vi "Configure.vi"(8 "error in":errorcluster, 10 "name":string="nCRDS", 11 "nCRD in":refnum<class "nCRD.lvclass">) -> (0 "error out":errorcluster, 3 "nCRD out":refnum<class "nCRD.lvclass">)   [LabVIEW 2015, in "nCRD.lvclass"]
doc: "Configures the CRDS for operation and starts all DAQmx tasks associated with the instrument. This VI overrides the parent VI in the Instrument class."
uses:
  nCRD.lvclass
  Reusable/Instrument/state.ctl
  Session/Raw FPGA/FPGA Session.lvclass
  nCRD.lvclass/nCRD.ctl
  Session/Raw FPGA/FPGA Session.lvclass/FPGA Session.ctl
  Reusable/Instrument/Instrument.lvclass/Instrument.ctl
  Session/Raw FPGA/Read FPGA Ref.vi
  Accessors/Write RepRate.vi
  Accessors/Write SamplesPerCycle.vi
  Reusable/Instrument/Read Log Session.vi
  <vilib>/Utility/error.llb/Error Cluster From Error Code.vi
  <vilib>/rvi/errors/niLvFpgaAdjustHostInterfaceError.vi
  Reusable/CRDS/Main/Read Cells.vi
  Reusable/CRDS/Cell/Write dt.vi
  Reusable/CRDS/Main/Write Cells.vi
  <vilib>/rvi/interface/common/niFpgaWaitOnOcc.vi
  FPGA Ref.ctl
  <vilib>/rvi/interface/nirviReadWriteControl/nirviReadWriteControl.xnode
  FPGA Bitfiles/NickIO.lvbitx
  Reusable/CRDS/Cell/CRDS Cell.lvclass
  <userlib>/_Session Fwk/Session - Root.lvclass
  <vilib>/rvi/interface/nirviMethod/nirviMethod.xnode
  Reusable/CRDS/Main/CRDS.lvclass
  <vilib>/rvi/errors/niLvFpgaMergeErrorWithErrorCode.vi
  Reusable/Instrument/Instrument.lvclass
  Reusable/Session Log/System Log.lvclass
  NiFpgaLv.dll
  <vilib>/FPGAPlugInAG/cRIO-9081/niLvFpga_ConfigureFifo_cRIO-9081.vi
  <vilib>/FPGAPlugInAG/cRIO-9081/niLvFpga_StartFifo_cRIO-9081.vi
panel:
  out "Actual Depth":u32
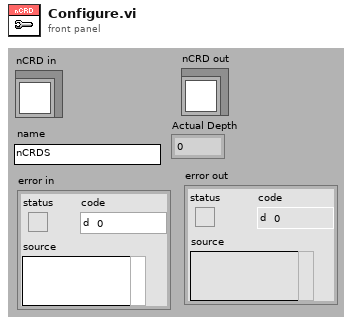
[diagram p1: front panel]
types:
  T1 = typedef "Instrument.lvclass/state.ctl" = enum8{"Configure", "Acquire", "Wait", "Quit", "Handle Error", "NOOP"}
  T2 = typedef "Session - Root.lvclass/Session Handle.ctl" = refnum<data-value>
  T3 = typedef "FPGA Ref.ctl" = refnum<k20>
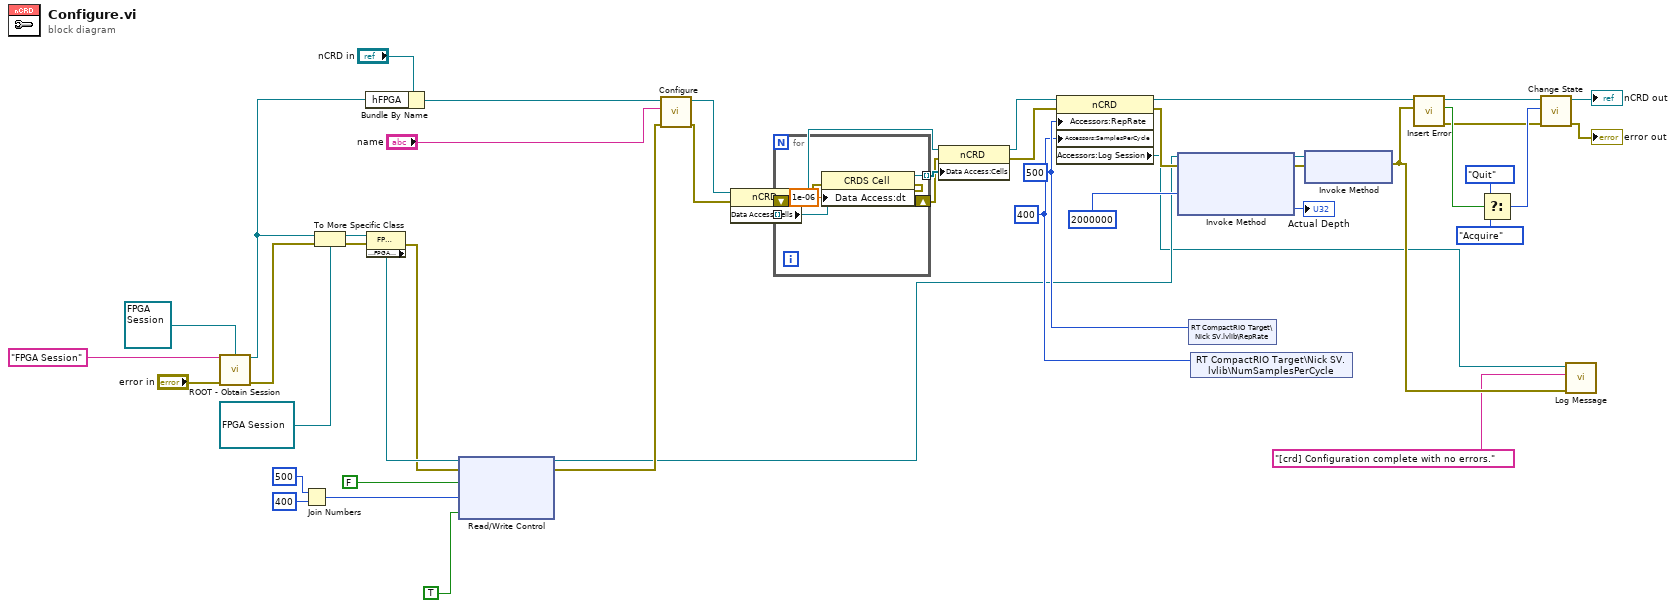
[diagram p0: block diagram]
diagram:
  w43 = u16 400 ("SamplesPerCycle")
  w44 = u16 500 ("RepRate")
  n1 = call <userlib>:"ROOT - Obtain Session.vi"("Session Name ()"="FPGA Session", "OBJ - Session"=refnum<class "FPGA Session.lvclass"> refnum ("FPGA Session.lvclass"), "error in (no error)"="error in") -> ("Session Handle"=w21:T2, "error out"=w20:errorcluster)  [unwired: 10 in, 1 out]
  n2 = Join Numbers(hi=u16 500 ("NumSamples"), lo=u16 400 ("DutyCycle")) -> ((hi.lo)=w1:u32)
  n3 = To More Specific Class(target class=refnum<data-value> refnum ("hFPGA"), reference=w21, error in=w20) -> (specific class reference=w28:refnum<data-value>, error out=w19:errorcluster)
  n4 = Bundle By Name(cluster="nCRD in", "hFPGA"=w21) -> (w22:refnum<class "nCRD.lvclass">)
  n5 = property class="FPGA Session"(reference=w28, error in=w19) -> (error out=w26:errorcluster, "Accessors:FPGA Ref"=w27:T3)  [unwired: 1 out]
  n6 = xnode "Read/Write Control"("FPGA VI Reference In"=w27, "error in"=w26, "Stop"=FALSE, "CRDSampData"=w1, "Transmit?"=TRUE) -> ("FPGA VI Reference Out"=w30:T3, "error out"=w31:errorcluster)
  n7 = call-parent "Configure.vi"("error in"=w31, "name"="name", "CRDS in"=w22) -> ("error out"=w12:errorcluster, "CRDS out"=w13:refnum<class "nCRD.lvclass">)  [unwired: 7 in]
  n8 = property class="nCRD"(reference=w13, error in=w12) -> (reference out=w9:refnum<class "nCRD.lvclass">, error out=w7:errorcluster, "Data Access:Cells"=w11:refnum<class "CRDS Cell.lvclass">[])
  n9 = for {
    tunnel: w11 -> [w53] mode=indexing
    tunnel: [w52] -> w10 mode=indexing
    shift-right: [w50] -> w6
    shift-left: w7 -> [w51]
    n10 = property class="CRDS Cell"(reference=w53, error in=w51, "Data Access:dt"=1e-06 ("dt")) -> (reference out=w52:refnum<class "CRDS Cell.lvclass">, error out=w50:errorcluster)
  }
  n11 = property class="nCRD"(reference=w9, error in=w6, "Data Access:Cells"=w10) -> (reference out=w8:refnum<class "nCRD.lvclass">, error out=w5:errorcluster)
  n12 = property class="nCRD"(reference=w8, error in=w5, "Accessors:RepRate"=w44, "Accessors:SamplesPerCycle"=w43) -> (reference out=w40:refnum<class "nCRD.lvclass">, error out=w45:errorcluster, "Accessors:Log Session"=w15:T2)
  n13 = xnode "Invoke Method"("FPGA VI Reference In"=w30, "error in"=w45, "Requested Depth"=u32 2000000) -> ("FPGA VI Reference Out"=w47:T3, "error out"=w46:errorcluster, "Actual Depth"=→"Actual Depth":u32)
  n14 = shared-variable "RT CompactRIO Target\\Nick SV.lvlib\\RepRate"(w44) -> ()  [unwired: 1 in, 1 out]
  n15 = shared-variable "RT CompactRIO Target\\Nick SV.lvlib\\NumSamplesPerCycle"(w43) -> ()  [unwired: 1 in, 1 out]
  n16 = xnode "Invoke Method"("FPGA VI Reference In"=w47, "error in"=w46) -> ("error out"=w16:errorcluster)  [unwired: 1 out]
  n17 = call "Insert Error.vi"("err"=w16, "Instrument in"=w40) -> ("error out"=w34:errorcluster, "error?"=w39:bool, "Instrument out"=w35:refnum<class "nCRD.lvclass">)  [unwired: 7 in]
  n18 = Select(t=state."Quit" ("instr state"), s=w39, f=state."Acquire" ("instr state")) -> (s? t:f=w38:T1)
  n19 = call "Change State.vi"("error in"=w34, "instr state"=w38, "Instrument in"=w35) -> ("error out"=→"error out":errorcluster, "Instrument out"=→"nCRD out":refnum<class "nCRD.lvclass">)  [unwired: 7 in]
  n20 = call "Log Message.vi"("error in"=w16, "MSG In"="[crd] Configuration complete with no errors.", "session in"=w15) -> ()  [unwired: 7 in, 2 out]
